vi "Clear Error.vi"(2 "Error In":errorcluster) -> (7 "no Error Out":errorcluster)   [LabVIEW 2019]
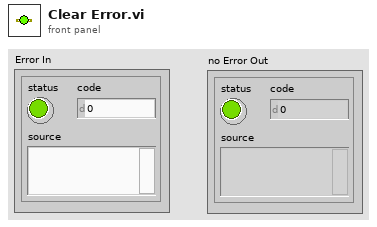
[diagram p1: front panel]
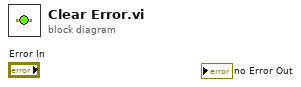
[diagram p0: block diagram]
diagram:
